vi "form clumps.vi"(8 "error in":errorcluster, 11 "clump precursors":T4[](array[typedef])) -> (0 "error out":errorcluster, 3 "clumps":T1[](array[typedef]))   [LabVIEW 2013, in "Modbus Module runtime.lvclass"]
uses:
  Modbus Module runtime.lvclass
  clump precursor.ctl
  module channel/data bank type.ctl
  <vilib>/NI/Tag Bus Module Framework/channel/channel classification.ctl
  clump accesses.ctl
  clump.ctl
  <vilib>/NI/Tag Bus Module Framework/channel/TBM channel.lvclass
  module channel/Modbus Module Channel.lvclass
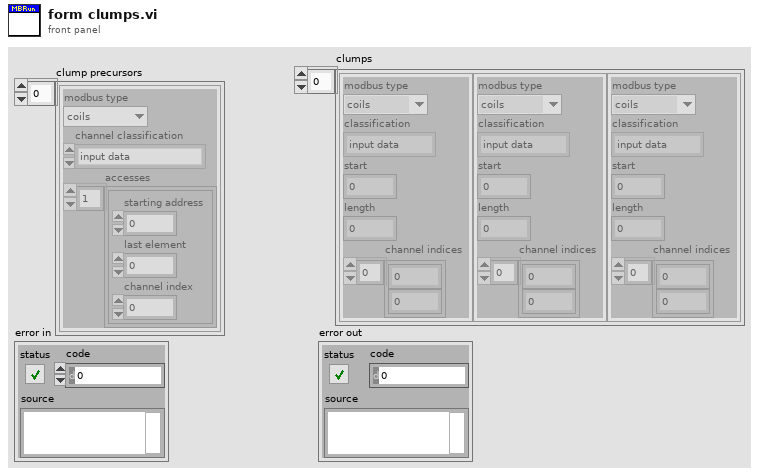
[diagram p1: front panel]
types:
  T1 = typedef "Modbus Module runtime.lvclass/clump.ctl" = cluster{"modbus type":T2, "classification":T3, "start":i32, "length":i32, "channel indices":i32[]}
  T2 = typedef "Modbus Module Channel.lvclass/data bank type.ctl" = enum16{"coils", "discrete inputs", "input registers", "holding registers"}
  T3 = typedef "TBM channel.lvclass/channel classification.ctl" = enum16{"input data", "output data", "processing parameter", "processing result"}
  T4 = typedef "Modbus Module runtime.lvclass/clump precursor.ctl" = cluster{"modbus type":T2, "channel classification":T3, "accesses":T5[]}
  T5 = typedef "Modbus Module runtime.lvclass/clump accesses.ctl" = cluster{"starting address":u16, "last element":i32, "channel index":i32}
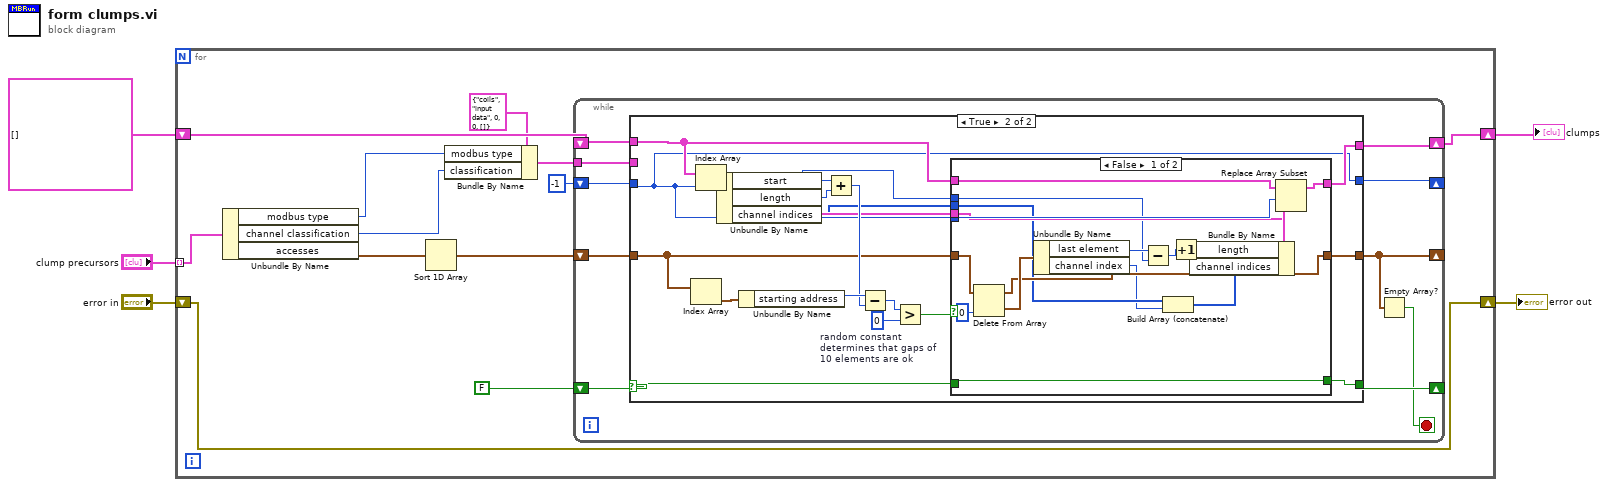
[diagram p0: block diagram]
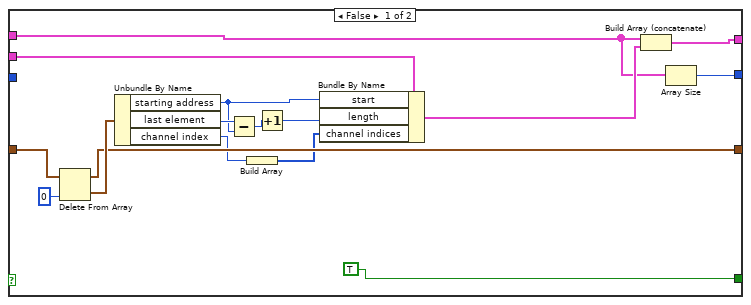
[diagram p2: hidden frame]
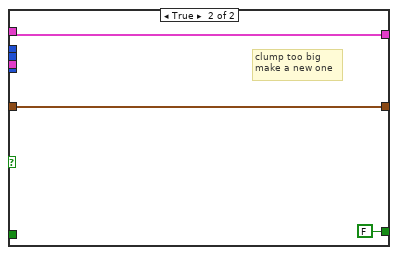
[diagram p3: hidden frame]
diagram:
  n1 = for {
    tunnel: "clump precursors" -> [w17] mode=indexing
    shift-right: [w6] -> w3
    shift-left: "error in" -> [w6]
    shift-right: [w14] -> w1
    shift-left: T1[] [] -> [w15]
    n2 = Unbundle By Name(w17) -> ("modbus type"=w11:T2, "channel classification"=w12:T3, "accesses"=w16:T5[])
    n3 = Sort 1D Array(array=w16) -> (sorted array=w10:T5[])
    n4 = Bundle By Name(cluster=T1 {"modbus type"=enum."coils", "classification"=enum."input data", "start"=0, "length"=0, "channel indices"=[]} ("output cluster"), "modbus type"=w11, "classification"=w12) -> (w9:T1)
    n5 = while {
      shift-right: [w22] -> _
      shift-left: w10 -> [w23]
      shift-right: [w24] -> w14
      shift-left: w15 -> [w25]
      shift-right: [w26] -> _
      shift-left: FALSE -> [w27]
      tunnel: w9 -> [w20]
      shift-right: [w18] -> _
      shift-left: -1 -> [w19]
      stop <- w21 stop-if-true
      n6 = case shown="True" w27 {
        selector: w27 -> [_ w53]
        tunnel: [TRUE w52] -> w26
        tunnel: w25 -> [w33 w49]
        tunnel: [w35 w48] -> w24
        tunnel: [w37 w51] -> w22
        tunnel: w23 -> [w43 w50]
        tunnel: w20 -> [w36 _]
        tunnel: w19 -> [_ w47]
        tunnel: [w32 w47] -> w18
        frame False {
          n7 = Delete From Array(array=w43, index=0) -> (deleted portion=w42:T5, array with subset deleted=w37:T5[])  [unwired: 1 in]
          n8 = Unbundle By Name(w42) -> ("starting address"=w40:u16, "last element"=w41:i32, "channel index"=w29:i32)
          n9 = Subtract(x=w41, y=w40) -> (x-y=w39:i32)
          n10 = Build Array(w29) -> (w28:i32[])
          n11 = Increment(x=w39) -> (x+1=w38:i32)
          n12 = Bundle By Name(cluster=w36, "start"=w40, "length"=w38, "channel indices"=w28) -> (w34:T1)
          n13 = Build Array (concatenate)(w33, w34) -> (w35:T1[])
          n14 = Array Size(array=w33) -> (size(s)=w32:i32)
        }
        frame True {
          w55 = 0  # random constant determines that gaps of 10 elements are ok
          n15 = Index Array(array=w50) -> (element=w59:T5)  [unwired: 1 in]
          n16 = Index Array(array=w49, index=w47) -> (element=w46:T1)
          n17 = Unbundle By Name(w46) -> ("start"=w45:i32, "length"=w60:i32, "channel indices"=w44:i32[])
          n18 = Unbundle By Name(w59) -> ("starting address"=w58:u16)
          n19 = Add(x=w45, y=w60) -> (x+y=w57:i32)
          n20 = Subtract(x=w58, y=w57) -> (x-y=w56:i32)
          n21 = Greater?(x=w56, y=w55) -> (0:w54:bool)
          n22 = case shown="False" w54 {
            tunnel: w53 -> [w66 _]
            tunnel: [w66 FALSE] -> w52
            tunnel: [w69 w80] -> w51
            tunnel: w50 -> [w70 w80]
            tunnel: w49 -> [w77 w79]
            tunnel: [w76 w79] -> w48
            tunnel: w47 -> [w75 _]
            tunnel: w46 -> [w67 _]
            tunnel: w45 -> [w65 _]
            tunnel: w44 -> [w63 _]
            frame False {
              n23 = Delete From Array(array=w70, index=0) -> (deleted portion=w74:T5, array with subset deleted=w69:T5[])  [unwired: 1 in]
              n24 = Unbundle By Name(w74) -> ("last element"=w73:i32, "channel index"=w62:i32)
              n25 = Subtract(x=w73, y=w65) -> (x-y=w72:i32)
              n26 = Build Array (concatenate)(w63, w62) -> (w61:i32[])
              n27 = Increment(x=w72) -> (x+1=w71:i32)
              n28 = Bundle By Name(cluster=w67, "length"=w71, "channel indices"=w61) -> (w68:T1)
              n29 = Replace Array Subset(array=w77, new element=w68, index=w75) -> (w76:T1[])
            }
            frame True {
              # "clump too big\nmake a new one"
            }
          }
        }
      }
      n30 = Empty Array?(array=w22) -> (empty?=w21:bool)
    }
  }
  "error out" <- w3
  "clumps" <- w1
